vi "DetachAndWritePosToQueue.vi"(8 "error in (no error)":errorcluster, 11 "XuLyStringUART in":refnum<class "XuLyStringUART.lvclass">) -> (0 "error out":errorcluster, 3 "XuLyStringUART out":refnum<class "XuLyStringUART.lvclass">)   [LabVIEW 2017, in "LibraryGcode.lvlib" / "XuLyStringUART.lvclass"]
uses:
  XuLyStringUART.lvclass
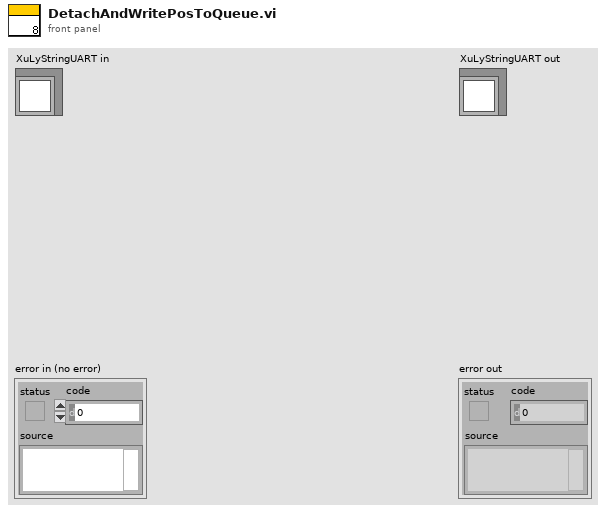
[diagram p1: front panel]
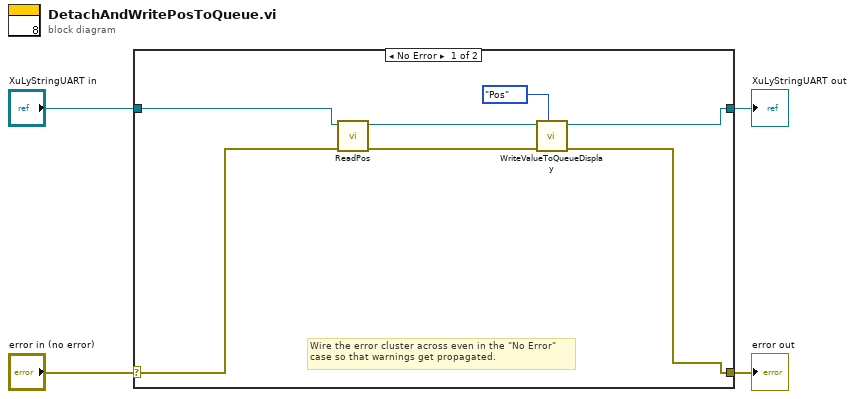
[diagram p0: block diagram]
diagram:
  n1 = case shown="No Error" "error in (no error)" {
    selector: "error in (no error)" -> [w10 w13]
    tunnel: [w6 w13] -> w3
    tunnel: [w7 w12] -> w1
    tunnel: "XuLyStringUART in" -> [w11 w12]
    frame No Error {
      # "Wire the error cluster across even in the \"No Error\"\ncase so that warnings get propagated."
      n2 = call-dynamic "ReadPos.vi"("error in (no error)"=w10, "XuLyStringUART in"=w11) -> ("error out"=w8:errorcluster, "XuLyStringUART out"=w9:refnum<class "XuLyStringUART.lvclass">)  [unwired: 8 in]
      n3 = call-dynamic "WriteValueToQueueDisplay.vi"("XuLyStringUART in"=w9, "error in (no error)"=w8, "Writepara"=enum16{"Config", "Pos"}."Pos") -> ("XuLyStringUART out"=w7:refnum<class "XuLyStringUART.lvclass">, "error out"=w6:errorcluster)  [unwired: 6 in]
    }
    frame Error {
    }
  }
  "error out" <- w3
  "XuLyStringUART out" <- w1
